vi "Untitled 1.vi"() -> ()   [LabVIEW 2024]
panel:
  out "x-y":u32
  out "value":u8
  in  "input parameter":u8
  in  "stop":bool
  out "CV Loop Time":u32=32
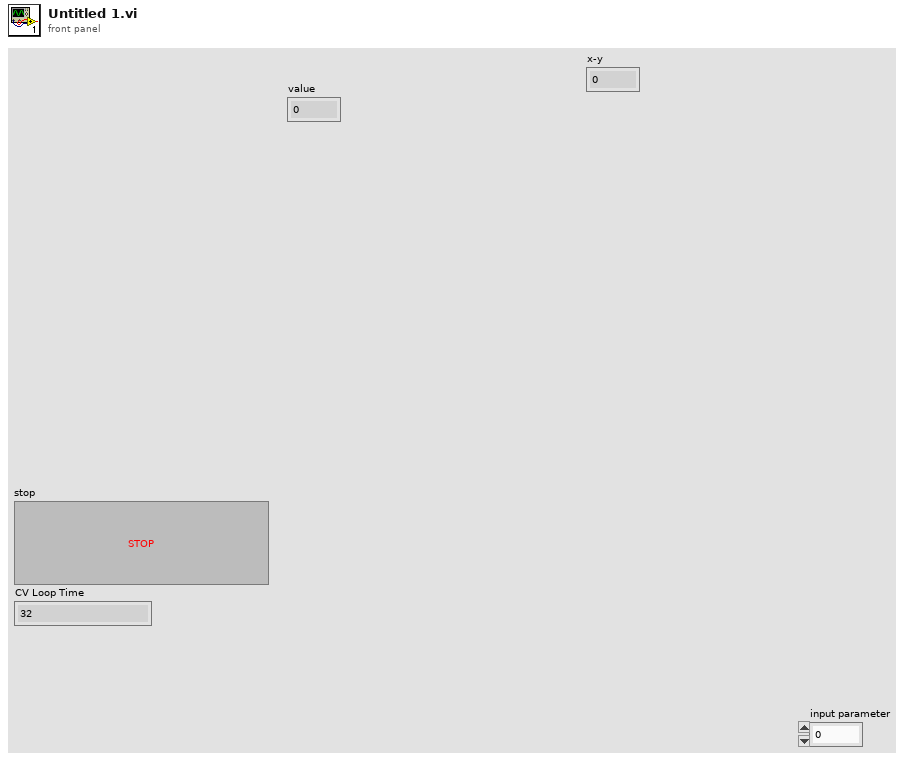
[diagram p1: front panel]
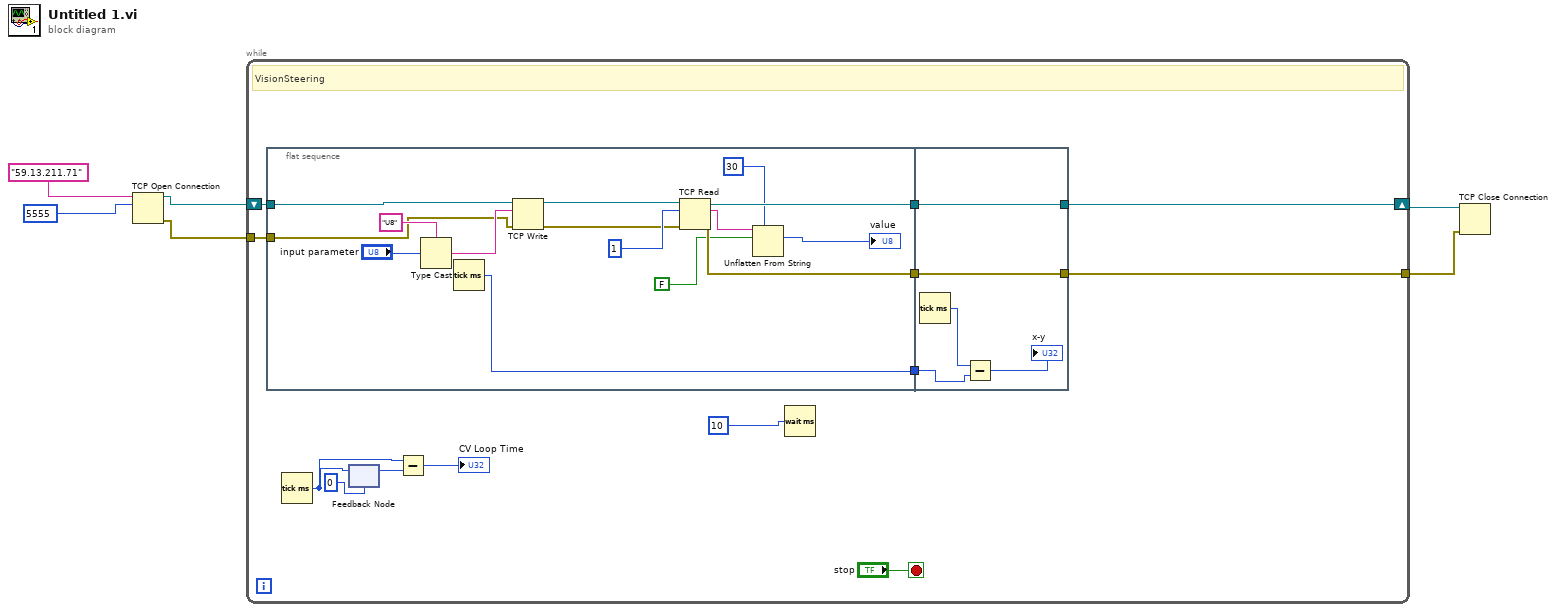
[diagram p0: block diagram]
diagram:
  n1 = TCP Open Connection(address="59.13.211.71", remote port or service name=u16 5555) -> (connection ID=w4:refnum<k5>, error out=w3:errorcluster)  [unwired: 3 in]
  n2 = while {
    tunnel: w3 -> [w13]
    tunnel: [w12] -> w2
    shift-right: [w10] -> w1
    shift-left: w4 -> [w14]
    stop <- "stop" stop-if-true
    # "VisionSteering"
    n3 = flat-sequence {
      tunnel: w14 -> [w34]
      tunnel: w13 -> [w30]
      tunnel: [w27] -> w9
      tunnel: [w25] -> w8
      tunnel: [w20] -> w7
      tunnel: [w38] -> w10
      tunnel: [w39] -> w12
      tunnel: w9 -> [w39]
      tunnel: w8 -> [w38]
      tunnel: w7 -> [w35]
      frame #0 {
        n4 = Type Cast(type="U8", x="input parameter") -> (*(type *) &x=w31:string)
        n5 = Tick Count (ms)() -> (millisecond timer value=w20:u32)
        n6 = TCP Write(connection ID=w34, data in=w31, error in (no error)=w30) -> (connection ID out=w29:refnum<k5>, error out=w26:errorcluster)  [unwired: 1 in, 1 out]
        n7 = TCP Read(connection ID=w29, bytes to read=1, error in (no error)=w26) -> (connection ID out=w25:refnum<k5>, data out=w24:string, error out=w27:errorcluster)  [unwired: 2 in]
        n8 = Unflatten From String(type=u8 30 ("input parameter 2"), binary string=w24, data includes array or string size? (T)=FALSE) -> (value=→"value":u8)  [unwired: 2 in, 2 out]
      }
      frame #1 {
        n9 = Tick Count (ms)() -> (millisecond timer value=w36:u32)
        n10 = Subtract(x=w36, y=w35) -> (x-y=→"x-y":u32)
      }
    }
    n11 = Tick Count (ms)() -> (millisecond timer value=w18:u32)
    n12 = feedback #1(u32 0 ("millisecond timer value")) -> (w17:u32)
    n13 = feedback-in #1(w18) -> ()
    n14 = Subtract(x=w18, y=w17) -> (x-y=→"CV Loop Time":u32)
    n15 = Wait (ms)(milliseconds to wait=u32 10) -> ()  [unwired: 1 out]
  }
  n16 = TCP Close Connection(connection ID=w1, error in (no error)=w2) -> ()  [unwired: 1 in, 2 out]
